vi "5492_Deadband.vi"(9 "Input":dbl, 10 "DeadBand":dbl) -> (1 "Output":dbl)   [LabVIEW 2016]
panel:
  # "Deadband should be positive"
  # "-1<= Input <= 1"
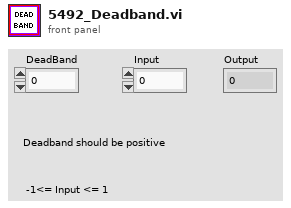
[diagram p1: front panel]
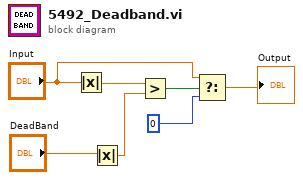
[diagram p0: block diagram]
diagram:
  n1 = Absolute Value(x="Input") -> (abs(x)=w3:dbl)
  n2 = Absolute Value(x="DeadBand") -> (abs(x)=w1:dbl)
  n3 = Greater?(x=w3, y=w1) -> (0:w7:bool)
  n4 = Select(t="Input", s=w7, f=0) -> (s? t:f=→"Output":dbl)
